vi "未命名 15.vi"(8 "error in":errorcluster caption="错误输入") -> (0 "error out":errorcluster caption="错误输出", 3 "task out":refnum<k21> caption="任务输出")   [LabVIEW 2020]
uses:
  <vilib>/DAQmx/create/channels.llb/DAQmx Create Channel (AO-Voltage-Basic).vi
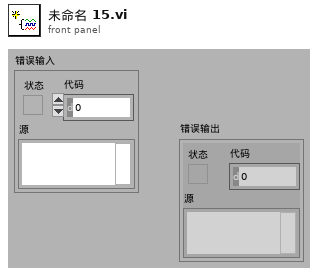
[diagram p1: front panel]
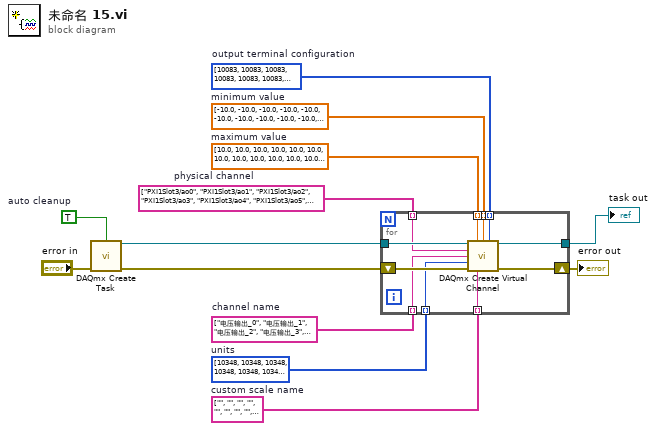
[diagram p0: block diagram]
diagram:
  w1 = i32[] [10083, 10083, 10083, 10083, 10083, 10083, 10083, 10083, 10083, 10083, 10083, 10083, 10083] items=["Default"=-1, "RSE"=10083, "Differential"=10106, "Pseudodifferential"=12529]  # output terminal configuration
  w7 = string[] ["", "", "", "", "", "", "", "", "", "", "", "", ""]  # custom scale name
  w6 = i32[] [10348, 10348, 10348, 10348, 10348, 10348, 10348, 10348, 10348, 10348, 10348, 10348, 10348] items=["Volts"=10348, "From Custom Scale"=10065]  # units
  w5 = string[] ["电压输出_0", "电压输出_1", "电压输出_2", "电压输出_3", "电压输出_4", "电压输出_5", "电压输出_6", "电压输出_7", "电压输出_8", "电压输出_9", "电压输出_10", "电压输出_11", "电压输出_12"]  # channel name
  w4 = string[] ["PXI1Slot3/ao0", "PXI1Slot3/ao1", "PXI1Slot3/ao2", "PXI1Slot3/ao3", "PXI1Slot3/ao4", "PXI1Slot3/ao5", "PXI1Slot3/ao6", "PXI1Slot3/ao7", "PXI1Slot3/ao8", "PXI1Slot3/ao9", "PXI1Slot3/ao10", "PXI1Slot3/ao11", "PXI1Slot3/ao12"]  # physical channel
  w8 = dbl[] [10.0, 10.0, 10.0, 10.0, 10.0, 10.0, 10.0, 10.0, 10.0, 10.0, 10.0, 10.0, 10.0]  # maximum value
  w9 = dbl[] [-10.0, -10.0, -10.0, -10.0, -10.0, -10.0, -10.0, -10.0, -10.0, -10.0, -10.0, -10.0, -10.0]  # minimum value
  w11 = TRUE  # auto cleanup
  n1 = call <vilib>:"DAQmx Create Task.vi"("auto cleanup"=w11, "error in"="error in") -> ("task out"=w10:refnum<k21>, "error out"=w12:errorcluster)  [unwired: 12 in]
  n2 = for "For循环" {
    tunnel: w10 -> [w22]
    tunnel: w9 -> [w23] mode=indexing
    tunnel: w8 -> [w24] mode=indexing
    tunnel: w7 -> [w15] mode=indexing
    tunnel: w6 -> [w16] mode=indexing
    tunnel: w5 -> [w18] mode=indexing
    tunnel: w4 -> [w17] mode=indexing
    tunnel: [w20] -> w3
    shift-right: [w19] -> w2
    shift-left: w12 -> [w21]
    tunnel: w1 -> [w14] mode=indexing
    n3 = call-poly <vilib>:"DAQmx Create Virtual Channel.vi"("task in"=w22, "maximum value"=w24, "minimum value"=w23, "output terminal configuration"=w14, "physical channels"=w17, "name to assign"=w18, "units"=w16, "error in"=w21, "custom scale name"=w15) -> ("task out"=w20:refnum<k21>, "error out"=w19:errorcluster)  [unwired: 5 in]
  }
  "error out" <- w2
  "task out" <- w3
